vi "UnLoadFrontEnd.vi"(8 "error in (no error)":errorcluster) -> (0 "error out":errorcluster, 3 "TestSetDef":T1={"General"={"ID"=0, "Model"="", "Dual Port?"=FALSE, "Options"="", "Options"={"E"=FALSE, "K"=FALSE, "H"=FALSE, "W"=FALSE, "F"=FALSE}, "Cal File"=path ""}, "Receiver"={"Fstart, MHz"=0.0, "Fstop MHz"=0.0, "Fstep MHz"=0.0, "IF, MHz"=0.0}, "RX Band"={"Fstart, MHz"=0.0, "Fstop MHz"=0.0}, "TX 1"={"Fstart, MHz"=0.0, "Fstop MHz"=0.0, "Pmax, dBm"=0.0, "Pstep, dB"=0.0}, "TX 2"={"Fstart, MHz"=0.0, "Fstop MHz"=0.0, "Pmax, dBm"=0.0, "Pstep, dB"=0.0}, "Low-side?"=TRUE})   [LabVIEW 2011]
uses:
  Test Set Definition.ctl
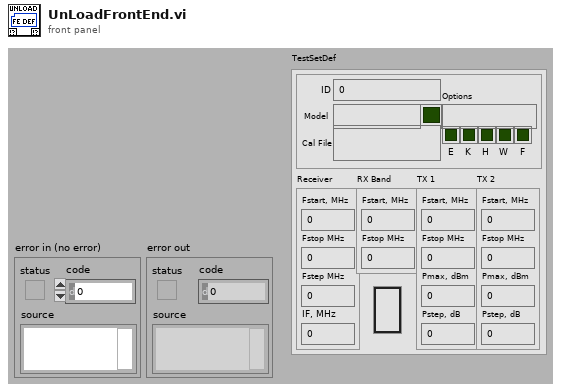
[diagram p1: front panel]
types:
  T1 = typedef "Test Set Definition.ctl" = cluster{"General":cluster{"ID":u32, "Model":string, "Dual Port?":bool, "Options":string, "Options":cluster{"E":bool, "K":bool, "H":bool, "W":bool, "F":bool}, "Cal File":path}, "Receiver":cluster{"Fstart, MHz":dbl, "Fstop MHz":dbl, "Fstep MHz":dbl, "IF, MHz":dbl}, "RX Band":cluster{"Fstart, MHz":dbl, "Fstop MHz":dbl}, "TX 1":cluster{"Fstart, MHz":dbl, "Fstop MHz":dbl, "Pmax, dBm":dbl, "Pstep, dB":dbl}, "TX 2":cluster{"Fstart, MHz":dbl, "Fstop MHz":dbl, "Pmax, dBm":dbl, "Pstep, dB":dbl}, "Low-side?":bool}
  T2 = cluster{"Command":string, "appended array":variant[]}
  T3 = cluster{"Command":string, "appended array":variant[]}[]
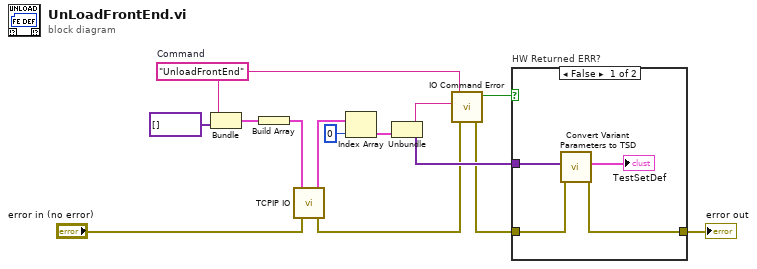
[diagram p0: block diagram]
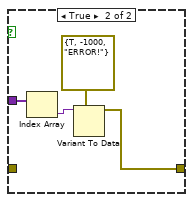
[diagram p2: hidden frame]
diagram:
  w11 = "UnloadFrontEnd"  # Command
  n1 = Bundle("Command"=w11, "appended array"=variant[] []) -> (w13:T2)  [unwired: 1 out]
  n2 = Build Array(w13) -> (w10:T3)
  n3 = call "TCPIP IO.vi"("error in (no error)"="error in (no error)", "Commands"=w10) -> ("error out"=w3:errorcluster, "Responses"=w9:cluster{string, variant[]}[])  [unwired: 1 in, 3 out]
  n4 = Index Array(array=w9, index=0) -> (element=w8:cluster{string, variant[]})
  n5 = Unbundle(w8) -> (w7:string, w5:variant[])
  n6 = call "IO Command Error.vi"("error in (no error)"=w3, "Command Returned (\"\")"=w7, "Command Sent (\"\")"=w11) -> ("error out"=w2:errorcluster, "HW ERR?"=w4:bool)  [unwired: 3 out]
  n7 = case "HW Returned ERR?" shown="False" w4 {
    tunnel: w2 -> [w16 _]
    tunnel: w5 -> [w18 w20]
    tunnel: [w15 w19] -> w1
    frame False {
      n8 = call "Convert Variant Parameters to TSD.vi"("error in"=w16, "Variant Parameter Array"=w18) -> ("error out"=w15:errorcluster, "TestSetDef"=→"TestSetDef":T1)  [unwired: 8 out]
    }
    frame True {
      n9 = Index Array(array=w20) -> (element=w22:variant)  [unwired: 1 in]
      n10 = Variant To Data(type=errorcluster {"status"=TRUE, "code"=-1000, "source"="ERROR!"} ("error out"), Variant=w22) -> (data=w19:errorcluster)  [unwired: 1 in, 1 out]
    }
  }
  "error out" <- w1
